vi "add.vi"(1 "Add Element":string, 2 "Buffer":string) -> (0 "New Buffer":string)   [LabVIEW 2018]
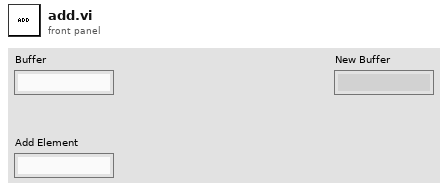
[diagram p1: front panel]
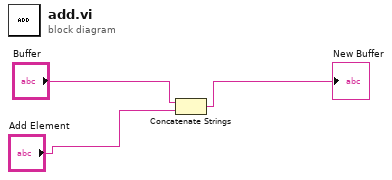
[diagram p0: block diagram]
diagram:
  n1 = Concatenate Strings("Buffer", "Add Element") -> (→"New Buffer":string)
